vi "Statistical_Measurements.vi"(1 "Array":dbl[][](array[numeric])) -> (0 "Dynamic Data":dynamicdata(waveform))   [LabVIEW 2023]
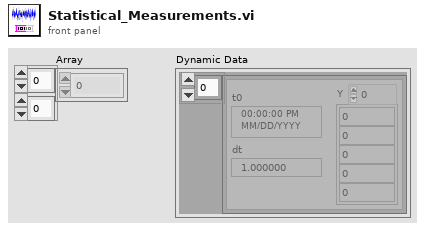
[diagram p1: front panel]
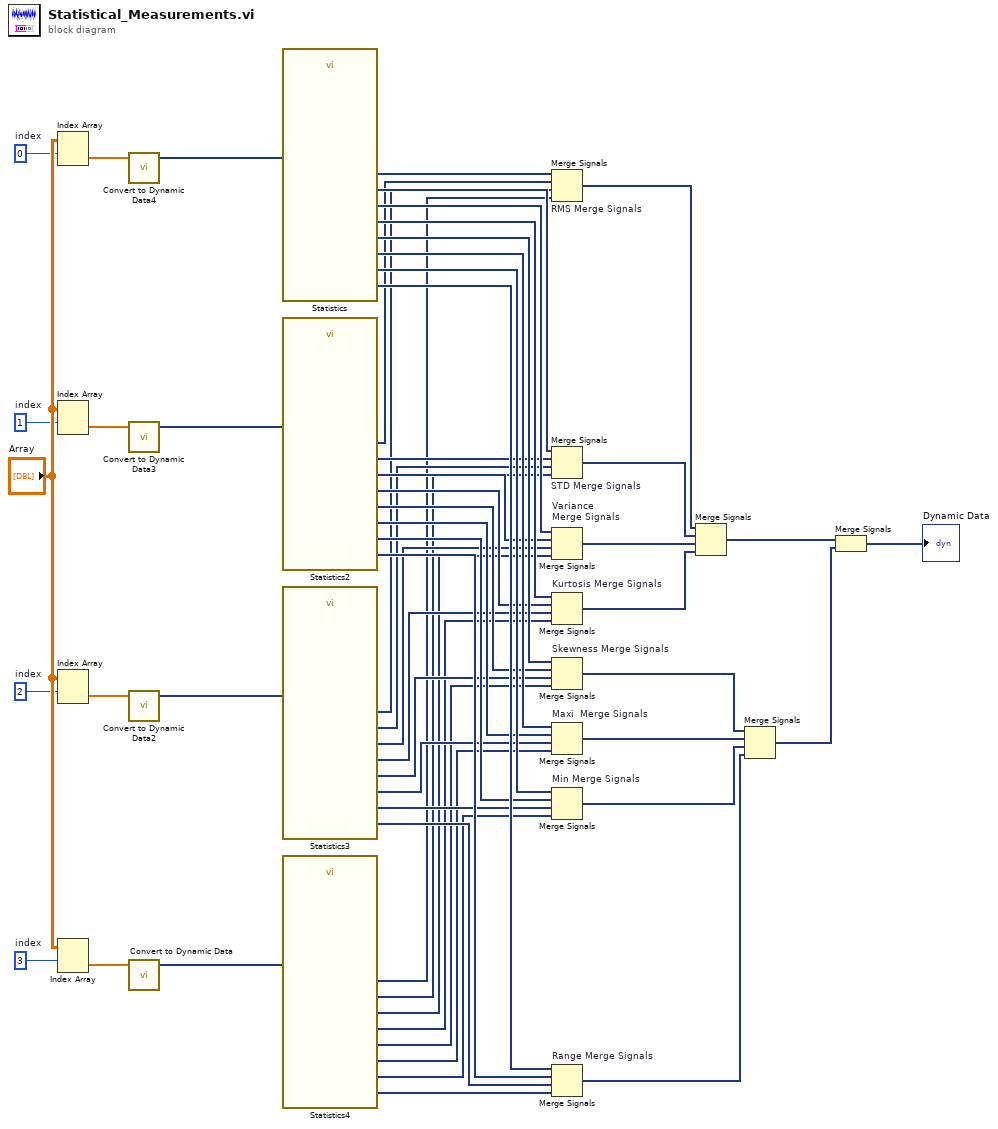
[diagram p0: block diagram]
diagram:
  w7 = 3  # index
  w5 = 2  # index
  w3 = 1  # index
  w1 = 0  # index
  n1 = Index Array "Index Array"(array="Array", index (row)=w1) -> (element=w2:dbl[])  [unwired: 1 in]
  n2 = Index Array "Index Array"(array="Array", index (row)=w3) -> (element=w4:dbl[])  [unwired: 1 in]
  n3 = Index Array "Index Array"(array="Array", index (row)=w5) -> (element=w6:dbl[])  [unwired: 1 in]
  n4 = Index Array "Index Array"(array="Array", index (row)=w7) -> (element=w8:dbl[])  [unwired: 1 in]
  n5 = call "Convert to Dynamic Data4"("Array"=w2) -> ("Dynamic Data Type"=w13:dynamicdata)  [unwired: 3 in]
  n6 = call "Convert to Dynamic Data3"("Array"=w4) -> ("Dynamic Data Type"=w12:dynamicdata)  [unwired: 3 in]
  n7 = call "Convert to Dynamic Data2"("Array"=w6) -> ("Dynamic Data Type"=w11:dynamicdata)  [unwired: 3 in]
  n8 = call "Convert to Dynamic Data"("Array"=w8) -> ("Dynamic Data Type"=w10:dynamicdata)  [unwired: 3 in]
  n9 = call "Statistics"("Signals"=w13) -> ("Skewness"=w41:dynamicdata, "Kurtosis"=w37:dynamicdata, "Variance"=w33:dynamicdata, "Standard Dev"=w29:dynamicdata, "RMS"=w25:dynamicdata, "Range"=w53:dynamicdata, "Minimum"=w49:dynamicdata, "Maximum"=w45:dynamicdata)  [unwired: 18 in, 1 out]
  n10 = call "Statistics2"("Signals"=w12) -> ("Skewness"=w42:dynamicdata, "Kurtosis"=w38:dynamicdata, "Variance"=w34:dynamicdata, "Standard Dev"=w30:dynamicdata, "RMS"=w26:dynamicdata, "Range"=w54:dynamicdata, "Minimum"=w50:dynamicdata, "Maximum"=w46:dynamicdata)  [unwired: 18 in, 1 out]
  n11 = call "Statistics3"("Signals"=w11) -> ("Skewness"=w43:dynamicdata, "Kurtosis"=w39:dynamicdata, "Variance"=w35:dynamicdata, "Standard Dev"=w31:dynamicdata, "RMS"=w27:dynamicdata, "Range"=w55:dynamicdata, "Minimum"=w51:dynamicdata, "Maximum"=w47:dynamicdata)  [unwired: 18 in, 1 out]
  n12 = call "Statistics4"("Signals"=w10) -> ("Skewness"=w44:dynamicdata, "Kurtosis"=w40:dynamicdata, "Variance"=w36:dynamicdata, "Standard Dev"=w32:dynamicdata, "RMS"=w28:dynamicdata, "Range"=w56:dynamicdata, "Minimum"=w52:dynamicdata, "Maximum"=w48:dynamicdata)  [unwired: 18 in, 1 out]
  n13 = Merge Signals "RMS Merge Signals"(w25, w26, w27, w28) -> (w16:dynamicdata)
  n14 = Merge Signals "STD Merge Signals"(w29, w30, w31, w32) -> (w17:dynamicdata)
  n15 = Merge Signals "Variance \nMerge Signals"(w33, w34, w35, w36) -> (w18:dynamicdata)
  n16 = Merge Signals "Kurtosis Merge Signals"(w37, w38, w39, w40) -> (w19:dynamicdata)
  n17 = Merge Signals "Skewness Merge Signals"(w41, w42, w43, w44) -> (w20:dynamicdata)
  n18 = Merge Signals "Maxi  Merge Signals"(w45, w46, w47, w48) -> (w21:dynamicdata)
  n19 = Merge Signals "Min Merge Signals"(w49, w50, w51, w52) -> (w22:dynamicdata)
  n20 = Merge Signals "Range Merge Signals"(w53, w54, w55, w56) -> (w23:dynamicdata)
  n21 = Merge Signals "Merge Signals"(w16, w17, w18, w19) -> (w15:dynamicdata)
  n22 = Merge Signals "Merge Signals"(w20, w21, w22, w23) -> (w24:dynamicdata)
  n23 = Merge Signals "Merge Signals"(w15, w24) -> (→"Dynamic Data":dynamicdata)
